vi "To Pretty String (String).vi"(7 "enable LabVIEW extensions? (T)":bool=TRUE, 8 "error in (no error)":errorcluster, 10 "indent":i32, 11 "JSON Value in":refnum<class "JSON Value.lvclass">) -> (0 "error out":errorcluster, 3 "String":string)   [LabVIEW 2016, in "JSON Value.lvclass"]
doc: "Flattens the given JSON data to a string."
uses:
  JSON Value.lvclass
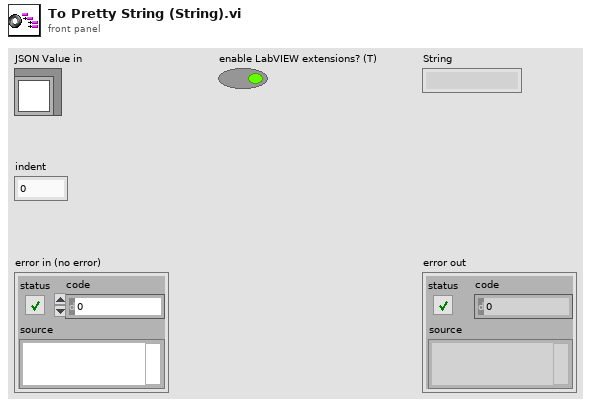
[diagram p1: front panel]
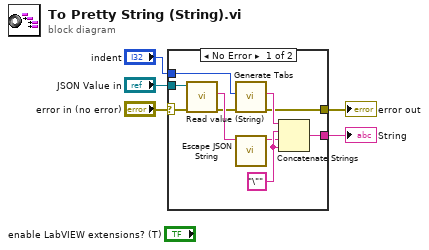
[diagram p0: block diagram]
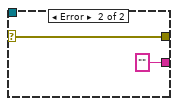
[diagram p2: hidden frame]
diagram:
  n1 = case shown="No Error" "error in (no error)" {
    selector: "error in (no error)" -> [w10 w16]
    tunnel: "JSON Value in" -> [w12 _]
    tunnel: [w14 ""] -> w4
    tunnel: [w6 w16] -> w3
    tunnel: "indent" -> [w9 _]
    frame No Error {
      w15 = "\"" ("string")
      n2 = call "Read value (String).vi"("error in (no error)"=w10, "JSON String in"=w12) -> ("error out"=w7:errorcluster, "value"=w11:string)  [unwired: 7 in, 1 out]
      n3 = call "Generate Tabs.vi"("error in (no error)"=w7, "indent"=w9) -> ("error out"=w6:errorcluster, "Tabs"=w8:string)  [unwired: 8 in]
      n4 = call "Escape JSON String.vi"("value"=w11) -> ("escaped string"=w13:string)  [unwired: 10 in]
      n5 = Concatenate Strings(w8, w15, w13, w15) -> (w14:string)
    }
    frame Error {
    }
  }
  "String" <- w4
  "error out" <- w3
